vi "Write Responder names.vi"(8 "error in (no error)":errorcluster, 10 "Responder names":string[](array[string]), 11 "Response Synchronizer in":refnum<class "Response Synchronizer.lvclass">) -> (0 "error out":errorcluster, 3 "Response Synchronizer out":refnum<class "Response Synchronizer.lvclass">)   [LabVIEW 2021, in "Response Synchronizer.lvclass"]
uses:
  Response Synchronizer.lvclass
  Response Synchronizer.lvclass/Response Synchronizer.ctl
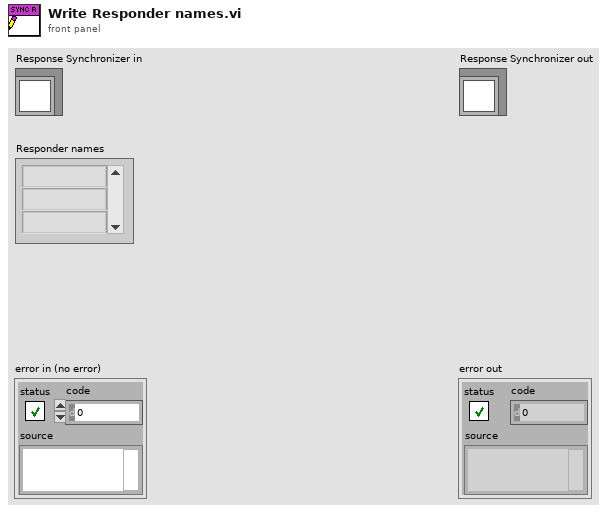
[diagram p1: front panel]
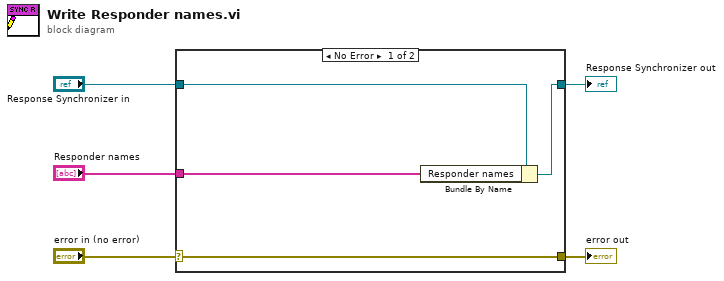
[diagram p0: block diagram]
diagram:
  n1 = case shown="No Error" "error in (no error)" {
    selector: "error in (no error)" -> [w9 w10]
    tunnel: [w9 w10] -> w4
    tunnel: [w7 w11] -> w2
    tunnel: "Response Synchronizer in" -> [w8 w11]
    tunnel: "Responder names" -> [w6 _]
    frame No Error {
      n2 = Bundle By Name(cluster=w8, "Responder names"=w6) -> (w7:refnum<class "Response Synchronizer.lvclass">)
    }
    frame Error {
    }
  }
  "error out" <- w4
  "Response Synchronizer out" <- w2
